vi "_Parse Measurement Response.vi"(0 "String In":string) -> (1 "Reliability":i32, 2 "Data":dbl[](array[numeric]) format="%^.3e")   [LabVIEW 2020, in "Rohde&Schwarz CMXP GPRF.lvlib"]
uses:
  <instrlib>/Rohde&Schwarz CMXP GPRF/Rohde&Schwarz CMXP GPRF.lvlib
  <instrlib>/Rohde&Schwarz CMXP GPRF/Private/rsidr_core.llb/rsidr_core.lvlib
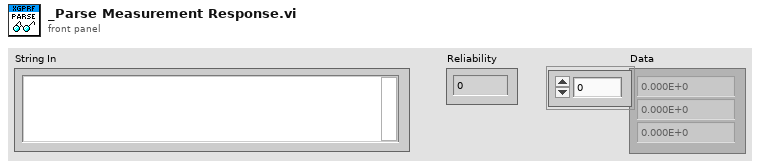
[diagram p1: front panel]
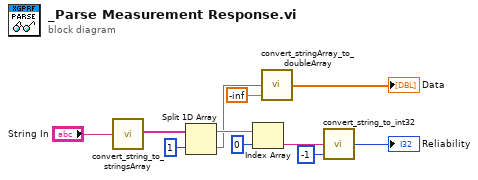
[diagram p0: block diagram]
diagram:
  n1 = call <instrlib>:"convert_string_to_stringsArray.vi"("String in"="String In") -> ("string array out"=w8:string[])  [unwired: 3 in, 1 out]
  n2 = Split 1D Array(array=w8, index=1) -> (first subarray=w6:string[], second subarray=w5:string[])
  n3 = Index Array(array=w6, index=0) -> (element=w3:string)
  n4 = call <instrlib>:"convert_stringArray_to_doubleArray.vi"("default (0)"=-inf ("Negative Infinity"), "string array in"=w5) -> ("double array out"=→"Data":dbl[])  [unwired: 3 in]
  n5 = call <instrlib>:"convert_string_to_int32.vi"("default (0)"=-1, "String in"=w3) -> ("int32 value out"=→"Reliability":i32)  [unwired: 3 in]
